vi "tester.vi"() -> ()   [LabVIEW 2017]
panel:
  in  "Boolean 2":bool
  out "bool":bool
  out "Output 01":dbl
  in  "Input 02":dbl
  in  "input 01":dbl
  out "Result message":string
  in  "Cluster 2":T1
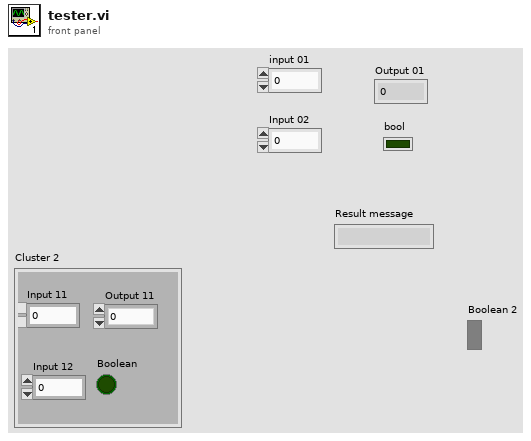
[diagram p1: front panel]
types:
  T1 = cluster{"Input 11":dbl, "Input 12":dbl, "Output 11":dbl, "Boolean":bool}
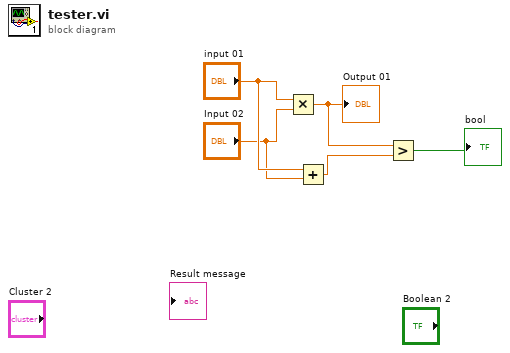
[diagram p0: block diagram]
diagram:
  n1 = Multiply(x="input 01", y="Input 02") -> (x*y=w3:dbl)
  "Output 01" <- w3
  n2 = Add(x="input 01", y="Input 02") -> (x+y=w2:dbl)
  n3 = Greater?(x=w3, y=w2) -> (0:→"bool":bool)
